vi "Chroma_PowerSupply_VoltSetting.vi"(8 "错误输入（无错误）":errorcluster, 10 "VoltageSetting":sgl, 11 "VISA资源名称":refnum<visa-resource-name>="COM1") -> (0 "错误输出":errorcluster, 3 "VISA资源名称输出":refnum<visa-resource-name>)   [LabVIEW 2012]
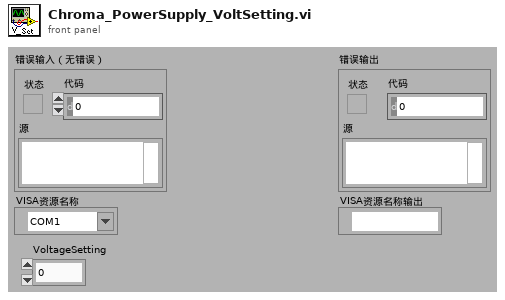
[diagram p1: front panel]
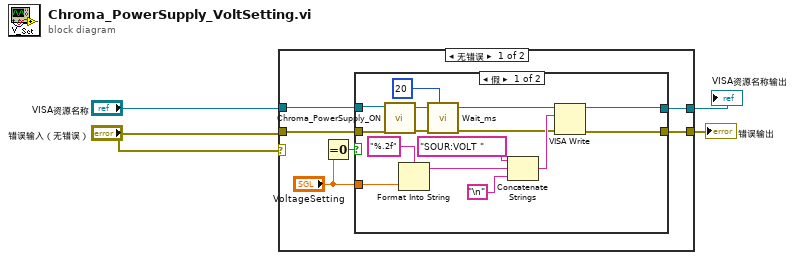
[diagram p0: block diagram]
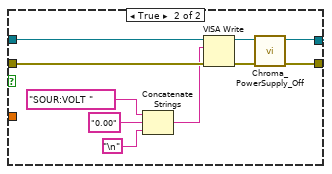
[diagram p2: hidden frame]
diagram:
  n1 = case shown="无错误" "错误输入（无错误）" {
    tunnel: "VISA资源名称" -> [w10 w36]
    tunnel: "错误输入（无错误）" -> [w9 w35]
    tunnel: [w8 w36] -> w4
    tunnel: [w7 w35] -> w3
    frame No Error {
      n2 = Equal To 0?(x="VoltageSetting") -> (x = 0?=w6:bool)
      n3 = case shown="假" w6 {
        tunnel: w10 -> [w18 w30]
        tunnel: w9 -> [w19 w26]
        tunnel: [w11 w33] -> w8
        tunnel: [w12 w34] -> w7
        tunnel: "VoltageSetting" -> [w13 _]
        frame False {
          n4 = call "Chroma_PowerSupply_ON.vi"("错误输入（无错误）"=w19, "VISA资源名称"=w18) -> ("错误输出"=w17:errorcluster, "VISA资源名称输出"=w15:refnum<visa-resource-name>)  [unwired: 8 out]
          n5 = Format Into String(format string="%.2f" ("格式字符串"), w13) -> (resulting string=w20:string)  [unwired: 2 in, 1 out]
          n6 = call "Wait_ms.vi"("等待时间（毫秒）"=u32 20, "错误输入（无错误）"=w17) -> ("error IO"=w16:errorcluster)  [unwired: 9 out]
          n7 = Concatenate Strings("SOUR:VOLT ", w20, "\n") -> (w23:string)
          n8 = VISA Write(VISA resource name=w15, write buffer=w23, error in (no error)=w16) -> (VISA resource name out=w11:refnum<visa-resource-name>, error out=w12:errorcluster)  [unwired: 1 out]
        }
        frame True {
          n9 = Concatenate Strings("SOUR:VOLT ", "0.00", "\n") -> (w25:string)
          n10 = VISA Write(VISA resource name=w30, write buffer=w25, error in (no error)=w26) -> (VISA resource name out=w31:refnum<visa-resource-name>, error out=w32:errorcluster)  [unwired: 1 out]
          n11 = call "Chroma_PowerSupply_Off.vi"("错误输入（无错误）"=w32, "VISA资源名称"=w31) -> ("错误输出"=w34:errorcluster, "VISA资源名称输出"=w33:refnum<visa-resource-name>)  [unwired: 8 out]
        }
      }
    }
    frame Error {
    }
  }
  "错误输出" <- w3
  "VISA资源名称输出" <- w4
